vi "_SampleQuery.vi"() -> ()   [LabVIEW 2013]
doc: "Example of how to do simple query using the driver library.\n\nNote the building of the instrument channel handle with the supplied vi, however for flexibility, the library will also interpret a plain integer string as being a GPIB address. (i.e. \"4\" will talk to GPIB address 4)"
panel:
  in  "GPIB Primary Address (4)":u8=4 min=1 max=31 step=1
  in  "Disable MAV check (F)":bool
  in  "Baud Rate (9600)":u32=9600 min=300 max=115200 step=300
  in  "COM Port (1)":u8=1 min=1 max=9 step=1
  in  "GPIB?":bool
  in  "stop":bool
  in  "Read":bool
  in  "Send":bool
  out "Response":string
  in  "Command to Write":string="R_B?"
  # "RS-232"
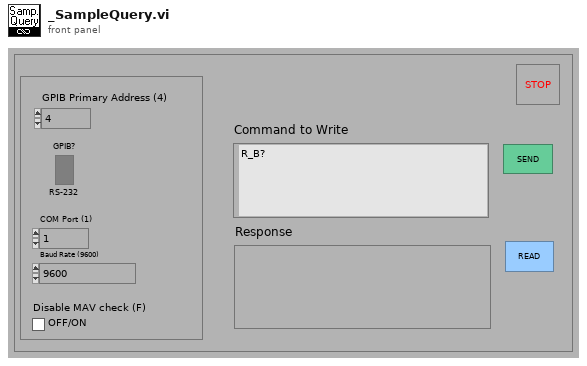
[diagram p1: front panel]
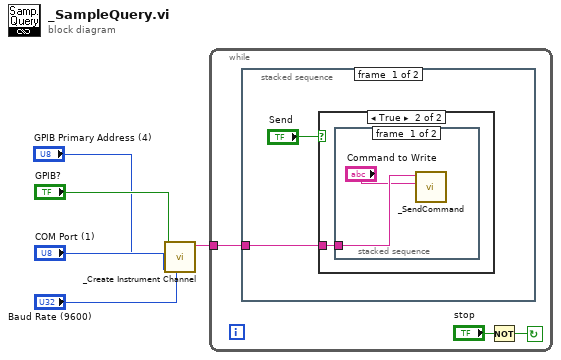
[diagram p0: block diagram]
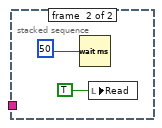
[diagram p3: hidden frame]
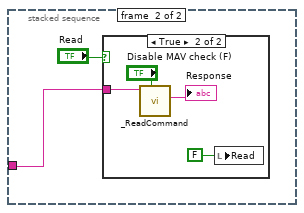
[diagram p4: hidden frame]
diagram:
  n1 = call "_Create Instrument Channel.vi"("Baud Rate (921600 - USB)"="Baud Rate (9600)", "COM Port (1)"="COM Port (1)", "GPIB Primary Address (4)"="GPIB Primary Address (4)", "(F), T - GPIB, F - RS232"="GPIB?") -> ("Instrument Channel out"=w2:string)  [unwired: 5 in, 2 out]
  n2 = while {
    tunnel: w2 -> [w6]
    stop <- w8 continue-if-true
    n3 = stacked-sequence {
      tunnel: w6 -> [w10 w17]
      frame #0 {
        n4 = case shown="True" "Send" {
          tunnel: w10 -> [_ w11]
          frame False {
          }
          frame True {
            n5 = stacked-sequence {
              tunnel: w11 -> [w13 _]
              frame #0 {
                n6 = call "_SendCommand.vi"("Command"="Command to Write", "Instrument Channel"=w13) -> ()  [unwired: 8 in, 2 out]
              }
              frame #1 {
                n7 = Wait (ms)(milliseconds to wait=50) -> ()  [unwired: 1 out]
                n8 = local write "Read"(TRUE) -> ()
              }
            }
          }
        }
      }
      frame #1 {
        n9 = case shown="True" "Read" {
          tunnel: w17 -> [_ w21]
          frame False {
          }
          frame True {
            n10 = call "_ReadCommand.vi"("Disable MAV check (F)"="Disable MAV check (F)", "Instrument Channel"=w21) -> ("Response"=→"Response":string)  [unwired: 7 in, 2 out]
            n11 = local write "Read"(FALSE) -> ()
          }
        }
      }
    }
    n12 = Not(x="stop") -> (.not. x?=w8:bool)
  }
